vi "_Cluster AutoSizing Dialog.vi"() -> (0 "cancelled?":bool=TRUE, 1 "Recursively (dup)":bool, 3 "type":T1(ring))   [LabVIEW 2012, in "Cluster AutoSizing.lvlib"]
uses:
  Cluster AutoSizing.lvlib
panel:
  in  "Recursively":bool
  in  "Arrange Veritcally":bool
  in  "Arrange Horizontally":bool
  in  "Size to fit":bool
  in  "None":bool
  # "1"
  # "2"
  # "3"
  # "4"
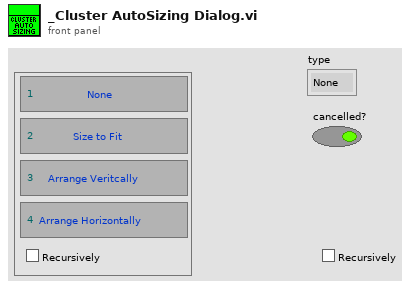
[diagram p1: front panel]
types:
  T1 = enum16{"None", "Size to Fit", "Arrange Horizontally", "Arrange Veritcally"}
  T2 = typedef "eventvkey.ctl" = enum16{"ASCII", "Enter", "Return", "Shift", "Ctrl", "Alt", "Cmd", "Opt", "Caps", "NumLock", "Clear", "Break", "Up", "Down", "Left", "Right", "Insert", "Delete", "Home", "End", "PageUp", "PageDown", "Escape", "Help", "Pause", "ScrollLock", "F1", "F2", "F3", "F4", "F5", "F6", "F7", "F8", "F9", "F10", "F11", "F12", "F13", "F14", "F15", "F16", "F17", "F18", "F19", "F20", "F21", "F22", "F23", "F24", "Play", "VolumeUp", "VolumeDown", "Mute", "Two Byte Char"}
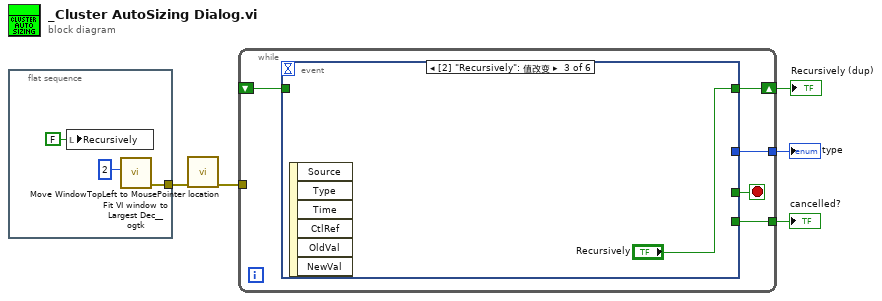
[diagram p0: block diagram]
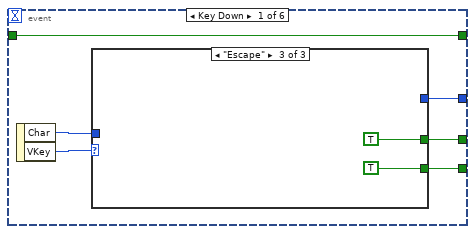
[diagram p2: hidden frame]
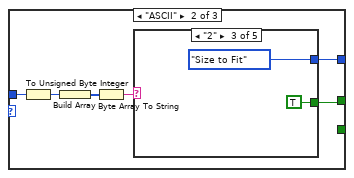
[diagram p4: hidden frame]
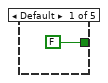
[diagram p5: hidden frame]
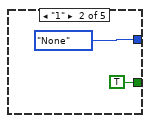
[diagram p6: hidden frame]
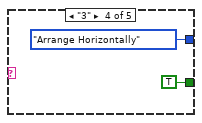
[diagram p7: hidden frame]
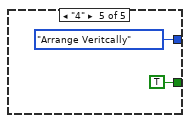
[diagram p8: hidden frame]
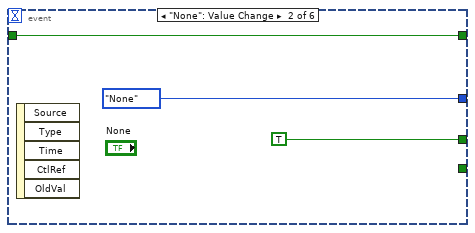
[diagram p9: hidden frame]
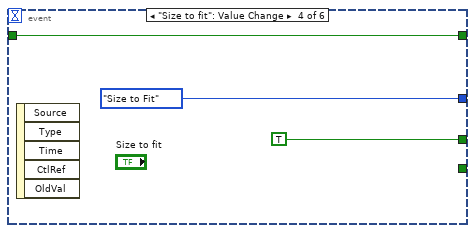
[diagram p10: hidden frame]
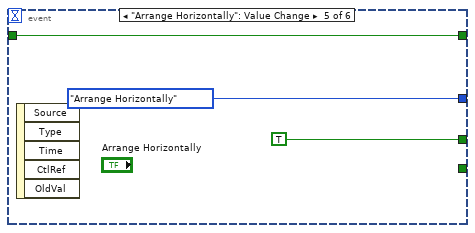
[diagram p11: hidden frame]
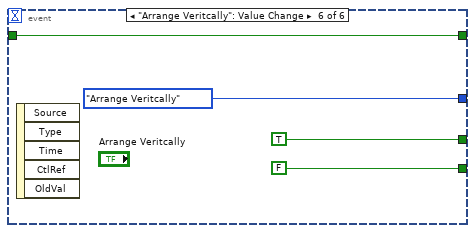
[diagram p12: hidden frame]
diagram:
  n1 = flat-sequence {
    tunnel: [w7] -> w1
    frame #0 {
      n2 = local write "Recursively"(FALSE ("Recursively")) -> ()
      n3 = call <userlib>:"Fit VI window to Largest Dec__ogtk.vi"("border spacing (2 px)"=2) -> ("error out"=w7:errorcluster)  [unwired: 5 in, 1 out]
    }
  }
  n4 = call "Move WindowTopLeft to MousePointer location.vi"("error in (no error)"=w1) -> ("error out"=w2:errorcluster)  [unwired: 10 in]
  n5 = while {
    tunnel: [w12] -> w4
    tunnel: [w11] -> w5
    shift-right: [w10] -> w3
    shift-left: _ -> [w9]
    tunnel: w2 -> [_]
    stop <- w13 stop-if-true
    n6 = event shown="[2] \"Recursively\": 值改变" {
      selector: _ -> [_ _ _ _ _ _]
      dyn-events: _ -> [_ _ _ _ _ _]
      timeout: _ -> [_ _ _ _ _ _]
      tunnel: [w18 TRUE _ TRUE TRUE TRUE] -> w13
      tunnel: [w17 _ _ _ _ FALSE] -> w12
      tunnel: [w15 T1."None" _ T1."Size to Fit" T1."Arrange Horizontally" T1."Arrange Veritcally"] -> w11
      tunnel: [w14 w37 "Recursively" w41 w44 w47] -> w10
      tunnel: w9 -> [w14 w37 _ w41 w44 w47]
      event Key Down {
        n7 = event-data() -> ("Char"=w16:i16, "VKey"=w19:T2)  [unwired: 1 in]
        n8 = case shown="\"Escape\"" w19 {
          tunnel: [_ w20 TRUE] -> w18
          tunnel: [_ _ TRUE] -> w17
          tunnel: w16 -> [_ w23 _]
          tunnel: [_ w21 _] -> w15
          frame Default {
          }
          frame "ASCII" {
            n9 = To Unsigned Byte Integer(number=w23) -> (unsigned 8bit integer=w24:u8)
            n10 = Build Array(w24) -> (w25:u8[])
            n11 = Byte Array To String(unsigned byte array=w25) -> (string=w22:string)
            n12 = case shown="\"2\"" w22 {
              tunnel: [_ T1."None" T1."Size to Fit" T1."Arrange Horizontally" T1."Arrange Veritcally"] -> w21
              tunnel: [FALSE TRUE TRUE TRUE TRUE] -> w20
              frame Default {
              }
              frame "1" {
              }
              frame "2" {
              }
              frame "3" {
              }
              frame "4" {
              }
            }
          }
          frame "Escape" {
          }
        }
      }
      event "None": Value Change {
        n13 = event-data() -> ()  [unwired: 1 in, 5 out]
      }
      event "Recursively": Value Change {
        n14 = event-data() -> ()  [unwired: 1 in, 6 out]
      }
      event "Size to fit": Value Change {
        n15 = event-data() -> ()  [unwired: 1 in, 5 out]
      }
      event "Arrange Horizontally": Value Change {
        n16 = event-data() -> ()  [unwired: 1 in, 5 out]
      }
      event "Arrange Veritcally": Value Change {
        n17 = event-data() -> ()  [unwired: 1 in, 5 out]
      }
    }
  }
  "type" <- w5
  "cancelled?" <- w4
  "Recursively (dup)" <- w3
